vi "Terminal-Alert-Handler.vi"(10 "开关":refnum<vi>, 11 "列表框":refnum<vi>) -> ()   [LabVIEW 2014]
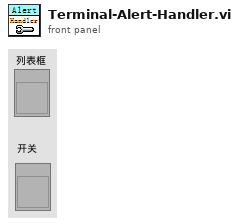
[diagram p1: front panel]
types:
  T1 = cluster{"报警级别":string, "报警系统":string, "报警详情":string, "备注":string}
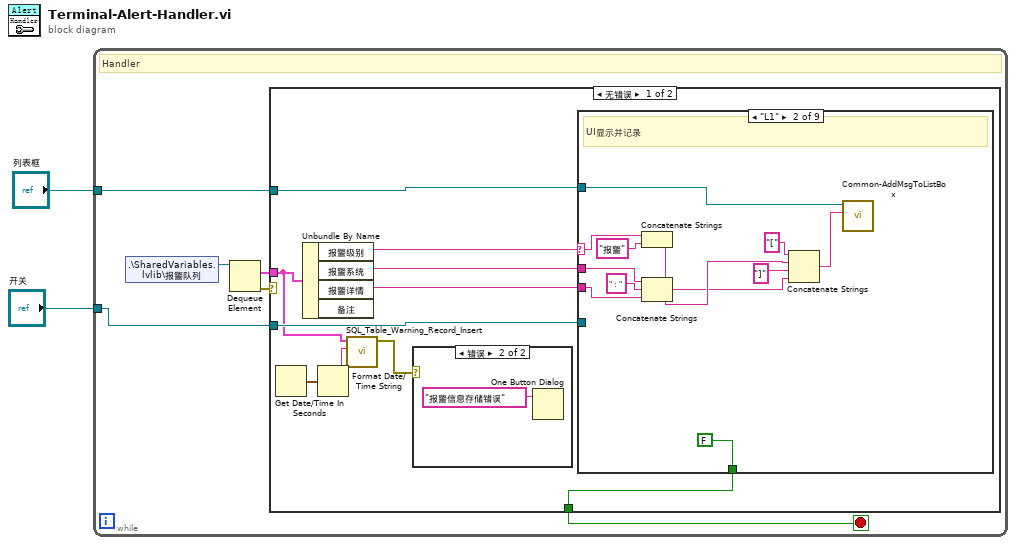
[diagram p0: block diagram]
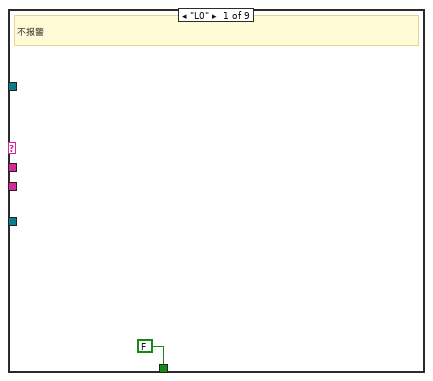
[diagram p3: hidden frame]
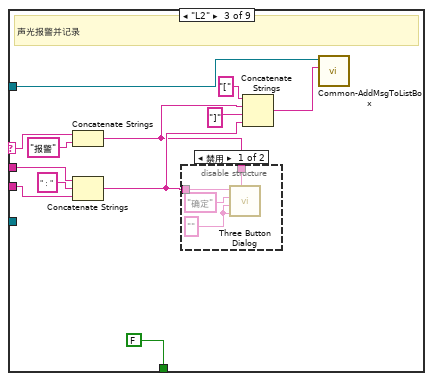
[diagram p4: hidden frame]
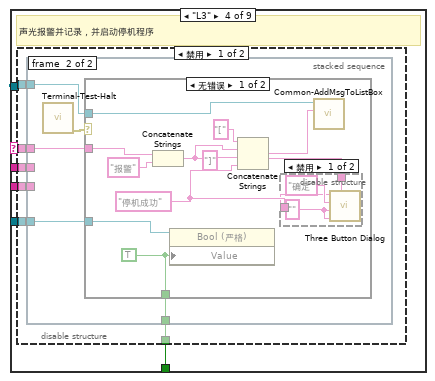
[diagram p6: hidden frame]
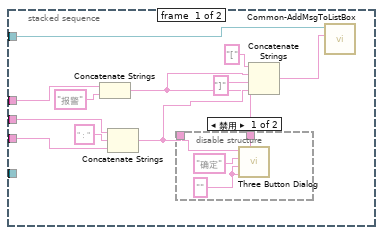
[diagram p7: hidden frame]
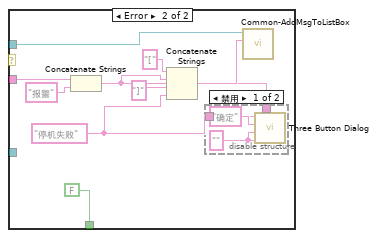
[diagram p10: hidden frame]
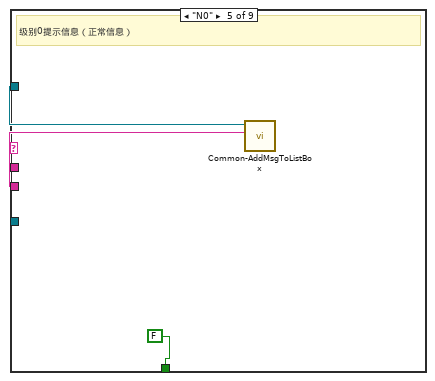
[diagram p13: hidden frame]
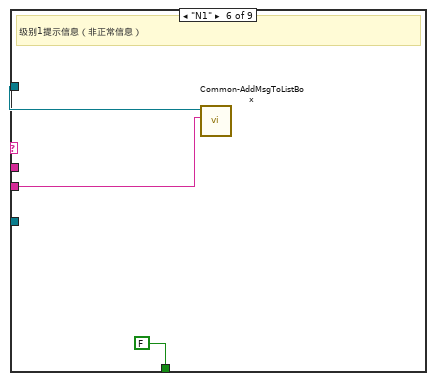
[diagram p14: hidden frame]
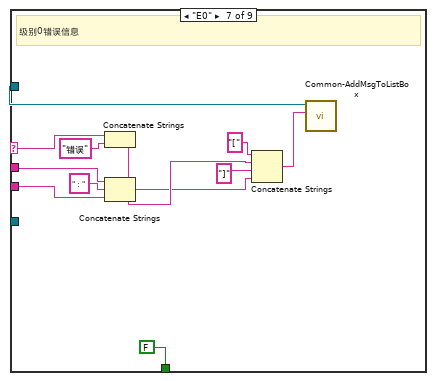
[diagram p15: hidden frame]
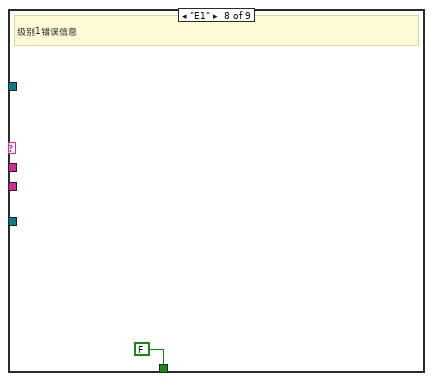
[diagram p16: hidden frame]
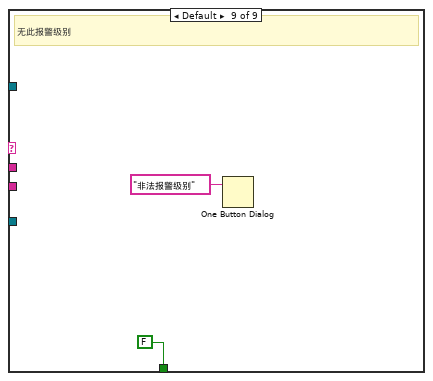
[diagram p17: hidden frame]
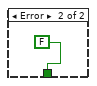
[diagram p18: hidden frame]
diagram:
  n1 = while {
    tunnel: "列表框" -> [w5]
    tunnel: "开关" -> [w4]
    stop <- w3 stop-if-true
    # "Handler"
    n2 = shared-variable ".\\SharedVariables.lvlib\\报警队列"() -> (w8:refnum<queue>)  [unwired: 1 in, 1 out]
    n3 = Dequeue Element(queue=w8) -> (element=w6:T1, error out=w7:errorcluster)  [unwired: 2 in, 2 out]
    n4 = case shown="无错误" w7 {
      tunnel: w6 -> [w11 _]
      tunnel: w5 -> [w15 _]
      tunnel: w4 -> [w14 _]
      tunnel: [w13 FALSE ("值")] -> w3
      frame No Error {
        n5 = Get Date/Time In Seconds() -> (seconds since 1Jan1904=w12:timestamp)
        n6 = Unbundle By Name(w11) -> ("报警级别"=w18:string, "报警系统"=w17:string, "报警详情"=w16:string)  [unwired: 1 out]
        n7 = Format Date/Time String(seconds (now)=w12) -> (date/time string=w10:string)  [unwired: 2 in]
        n8 = call "SQL_Table_Warning_Record_Insert.vi"("时间"=w10, "报警信息"=w11) -> ("error out"=w9:errorcluster)  [unwired: 9 in]
        n9 = case shown="错误" w9 {
          frame No Error {
          }
          frame Error {
            n10 = One Button Dialog(message="报警信息存储错误" ("消息")) -> ()  [unwired: 1 in, 1 out]
          }
        }
        n11 = case shown="\"L1\"" w18 {
          selector: w18 -> [_ w29 w40 w52 _ _ w116 _ _]
          tunnel: w17 -> [_ w32 w43 w54 _ _ w115 _ _]
          tunnel: w16 -> [_ w30 w42 w53 w108 w111 w114 _ _]
          tunnel: w15 -> [_ w27 w34 w51 w109 w112 w117 _ _]
          tunnel: w14 -> [_ _ _ w50 _ _ _ _ _]
          tunnel: [FALSE ("值") FALSE ("值") FALSE ("值") w49 FALSE ("值") FALSE ("值") FALSE ("值") FALSE ("值") FALSE ("值")] -> w13
          frame "L0" {
            # "不报警"
          }
          frame "L1" {
            # "UI显示并记录"
            n12 = Concatenate Strings(w29, "报警" ("字符串")) -> (w24:string)
            n13 = Concatenate Strings(w32, "：" ("字符串"), w30) -> (w21:string)
            n14 = Concatenate Strings("[" ("字符串"), w24, "]" ("字符串"), w21) -> (w23:string)
            n15 = call "Common-AddMsgToListBox.vi"("字符串"=w23, "列表框"=w27) -> ()  [unwired: 10 in]
          }
          frame "L2" {
            # "声光报警并记录"
            n16 = Concatenate Strings(w40, "报警" ("字符串")) -> (w35:string)
            n17 = Concatenate Strings(w43, "：" ("字符串"), w42) -> (w36:string)
            n18 = disable-structure shown="禁用" {
              disable-tunnel: w36 -> [w46 _]
              disable-tunnel: w35 -> [w45 _]
              frame Disabled {
                w48 = "" ("Center Button Text (\"No\")")
                n19 = call <vilib>:"Three Button Dialog.vi"("Window Title (\"\")"=w45, "Right Button Text (\"Cancel\")"=w48, "Center Button Text (\"No\")"=w48, "Left Button Text (\"Yes\")"="确定" ("Left Button Text (\"Yes\")"), "message"=w46) -> ()  [unwired: 6 in, 1 out]
              }
              frame Enabled {
              }
            }
            n20 = Concatenate Strings("[" ("字符串"), w35, "]" ("字符串"), w36) -> (w37:string)
            n21 = call "Common-AddMsgToListBox.vi"("字符串"=w37, "列表框"=w34) -> ()  [unwired: 10 in]
          }
          frame "L3" {
            # "声光报警并记录，并启动停机程序"
            n22 = disable-structure shown="禁用" {
              disable-tunnel: w54 -> [w60 _]
              disable-tunnel: w53 -> [w59 _]
              disable-tunnel: w52 -> [w58 _]
              disable-tunnel: w51 -> [w57 _]
              disable-tunnel: w50 -> [w56 _]
              disable-tunnel: [w55 _] -> w49
              frame Disabled {
                n23 = stacked-sequence {
                  tunnel: w60 -> [w69 _]
                  tunnel: w59 -> [w68 _]
                  tunnel: w58 -> [w67 w79]
                  tunnel: w57 -> [w61 w78]
                  tunnel: w56 -> [_ w77]
                  tunnel: [_ w76] -> w55
                  frame #0 {
                    n24 = Concatenate Strings(w67, "报警" ("字符串")) -> (w62:string)
                    n25 = Concatenate Strings(w69, "：" ("字符串"), w68) -> (w63:string)
                    n26 = disable-structure shown="禁用" {
                      disable-tunnel: w63 -> [w73 _]
                      disable-tunnel: w62 -> [w72 _]
                      frame Disabled {
                        w75 = "" ("Center Button Text (\"No\")")
                        n27 = call <vilib>:"Three Button Dialog.vi"("Window Title (\"\")"=w72, "Right Button Text (\"Cancel\")"=w75, "Center Button Text (\"No\")"=w75, "Left Button Text (\"Yes\")"="确定" ("Left Button Text (\"Yes\")"), "message"=w73) -> ()  [unwired: 6 in, 1 out]
                      }
                      frame Enabled {
                      }
                    }
                    n28 = Concatenate Strings("[" ("字符串"), w62, "]" ("字符串"), w63) -> (w64:string)
                    n29 = call "Common-AddMsgToListBox.vi"("字符串"=w64, "列表框"=w61) -> ()  [unwired: 10 in]
                  }
                  frame #1 {
                    n30 = call "Terminal-Test-Halt.vi"() -> ("error out"=w80:errorcluster)  [unwired: 11 in]
                    n31 = case shown="无错误" w80 {
                      tunnel: w79 -> [w89 w102]
                      tunnel: w78 -> [w83 w96]
                      tunnel: w77 -> [w82 _]
                      tunnel: [w81 FALSE ("值")] -> w76
                      frame No Error {
                        w81 = TRUE ("值")
                        w85 = "停机成功" ("消息")
                        n32 = Concatenate Strings(w89, "报警" ("字符串")) -> (w84:string)
                        n33 = property class="Bool (严格)"(reference=w82, "Value"=w81) -> ()  [unwired: 1 in, 2 out]
                        n34 = Concatenate Strings("[" ("字符串"), w84, "]" ("字符串"), w85) -> (w86:string)
                        n35 = disable-structure shown="禁用" {
                          disable-tunnel: w85 -> [w92 _]
                          disable-tunnel: w84 -> [w91 _]
                          frame Disabled {
                            w94 = "" ("Center Button Text (\"No\")")
                            n36 = call <vilib>:"Three Button Dialog.vi"("Window Title (\"\")"=w91, "Right Button Text (\"Cancel\")"=w94, "Center Button Text (\"No\")"=w94, "Left Button Text (\"Yes\")"="确定" ("Left Button Text (\"Yes\")"), "message"=w92) -> ()  [unwired: 6 in, 1 out]
                          }
                          frame Enabled {
                          }
                        }
                        n37 = call "Common-AddMsgToListBox.vi"("字符串"=w86, "列表框"=w83) -> ()  [unwired: 10 in]
                      }
                      frame Error {
                        w98 = "停机失败" ("消息")
                        n38 = Concatenate Strings(w102, "报警" ("字符串")) -> (w97:string)
                        n39 = Concatenate Strings("[" ("字符串"), w97, "]" ("字符串"), w98) -> (w99:string)
                        n40 = disable-structure shown="禁用" {
                          disable-tunnel: w98 -> [w105 _]
                          disable-tunnel: w97 -> [w104 _]
                          frame Disabled {
                            w107 = "" ("Center Button Text (\"No\")")
                            n41 = call <vilib>:"Three Button Dialog.vi"("Window Title (\"\")"=w104, "Right Button Text (\"Cancel\")"=w107, "Center Button Text (\"No\")"=w107, "Left Button Text (\"Yes\")"="确定" ("Left Button Text (\"Yes\")"), "message"=w105) -> ()  [unwired: 6 in, 1 out]
                          }
                          frame Enabled {
                          }
                        }
                        n42 = call "Common-AddMsgToListBox.vi"("字符串"=w99, "列表框"=w96) -> ()  [unwired: 10 in]
                      }
                    }
                  }
                }
              }
              frame Enabled {
              }
            }
          }
          frame "N0" {
            # "级别0提示信息（正常信息）"
            n43 = call "Common-AddMsgToListBox.vi"("字符串"=w108, "列表框"=w109) -> ()  [unwired: 10 in]
          }
          frame "N1" {
            # "级别1提示信息（非正常信息）"
            n44 = call "Common-AddMsgToListBox.vi"("字符串"=w111, "列表框"=w112) -> ()  [unwired: 10 in]
          }
          frame "E0" {
            # "级别0错误信息"
            n45 = Concatenate Strings(w116, "错误" ("字符串")) -> (w120:string)
            n46 = Concatenate Strings(w115, "：" ("字符串"), w114) -> (w118:string)
            n47 = Concatenate Strings("[" ("字符串"), w120, "]" ("字符串"), w118) -> (w119:string)
            n48 = call "Common-AddMsgToListBox.vi"("字符串"=w119, "列表框"=w117) -> ()  [unwired: 10 in]
          }
          frame "E1" {
            # "级别1错误信息"
          }
          frame Default {
            # "无此报警级别"
            n49 = One Button Dialog(message="非法报警级别" ("消息")) -> ()  [unwired: 1 in, 1 out]
          }
        }
      }
      frame Error {
      }
    }
  }
